vi "test TDMS.vi"   [LabVIEW 2013]
uses:
  <vilib>/addons/Electrical Power/Basic/NI_EP_Basic.lvlib
  <vilib>/addons/Electrical Power/Basic/Measurement/RMS (N Channels).vi
types:
  T1 = typedef "Test Case.ctl" = cluster{"Lamp":string, "Transformer":string, "Dimmer":string, "Dim Level":string, "Lamp Number":string}
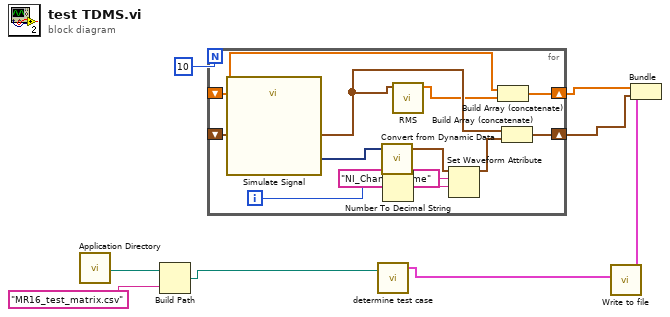
[diagram p0: block diagram]
diagram:
  n1 = call <vilib>:"Application Directory.vi"() -> ("Application Directory"=w7:path)
  n2 = Build Path(base path=w7, name or relative path="MR16_test_matrix.csv") -> (appended path=w6:path)
  n3 = for {
    N: 10 -> [_]
    shift-right: [w19] -> w2
    shift-left: _ -> [w12]
    shift-right: [w10] -> w3
    shift-left: _ -> [w9]
    i -> [w15]
    n4 = call "Simulate Signal"() -> ("Sine"=w18:dynamicdata)  [unwired: 14 in, 1 out]
    n5 = call "Convert from Dynamic Data"("Dynamic Data Type"=w18) -> ("Waveform"=w17:waveform(dbl))  [unwired: 3 in]
    n6 = Number To Decimal String(number=w15) -> (decimal integer string=w14:string)  [unwired: 1 in]
    n7 = call-poly <vilib>:"RMS.vi"("waveforms"=w12) -> ("RMS values"=w11:dbl[])  [unwired: 9 in, 1 out]
    n8 = Set Waveform Attribute(5:w14, 6:"NI_ChannelName" ("name"), 7:w17) -> (3:w16:waveform(dbl))  [unwired: 1 in, 2 out]
    n9 = Build Array (concatenate)(w9, w11) -> (w10:dbl[])
    n10 = Build Array (concatenate)(w12, w16) -> (w19:waveform(dbl)[])
  }
  n11 = call "determine test case.vi"("file path (dialog if empty)"=w6) -> ("Test Case Cluster"=w5:T1)  [unwired: 1 in, 2 out]
  n12 = Bundle(w3, w2) -> (w1:cluster{dbl[], waveform(dbl)[]})  [unwired: 1 in]
  n13 = call "Write to file.vi"("Test Case"=w5, "Don't wait for stabilizatoin"=w1) -> ()  [unwired: 9 in, 1 out]
